vi "Test Message in Ressult without Description.vi"(8 "error in (no error)":errorcluster, 11 "Compare Assertion Test In":refnum<class "Compare Assertion Test.lvclass">) -> (0 "error out":errorcluster, 3 "Compare Assertion Test Out":refnum<class "Compare Assertion Test.lvclass">)   [LabVIEW 2020, in "LUnit Tests.lvlib" / "Compare Assertion Test.lvclass"]
uses:
  Compare Assertion Test.lvclass
  Compare Assertion Test.lvclass/Compare Assertion Test.ctl
  Test Dummys/Test Case Test Double/Test Case Test Double.lvclass
  <vilib>/Astemes/LUnit/Test Case.lvclass
  C:/Program Files (x86)/National Instruments/LabVIEW 2020/vi.lib/Astemes/LUnit/Test Case.lvclass
  C:/Git/astemes-lunit/tests/Compare Assertion Test/Compare Assertion Test.lvclass
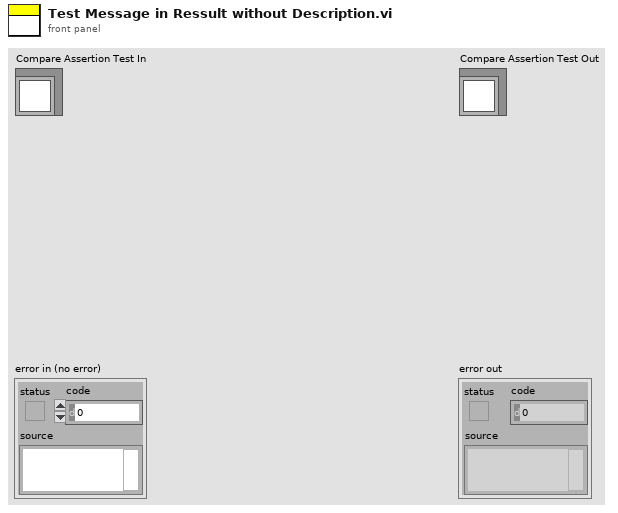
[diagram p1: front panel]
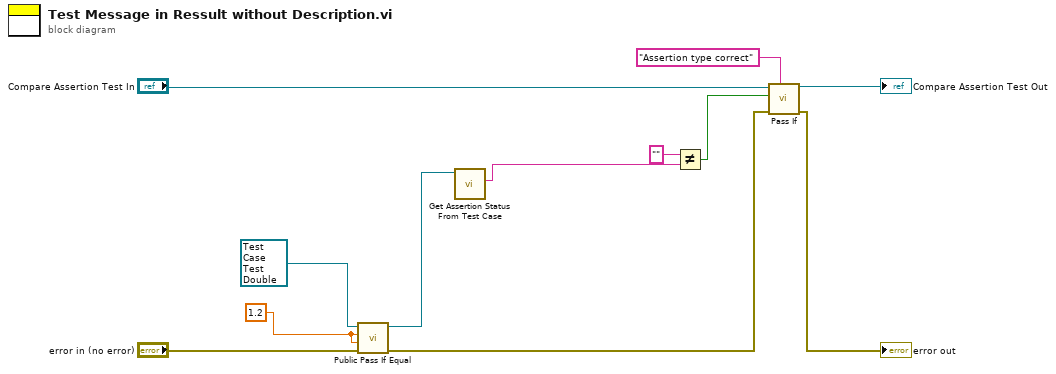
[diagram p0: block diagram]
diagram:
  w3 = 1.2
  n1 = call "Public Pass If Equal.vi"("error in (no error)"="error in (no error)", "Actual"=w3, "Expected"=w3, "Test Case Test Double in"=refnum<class "Test Case Test Double.lvclass"> refnum ("Test Case Test Double.lvclass")) -> ("error out"=w9:errorcluster, "Test Case Test Double out"=w8:refnum<class "Test Case Test Double.lvclass">)  [unwired: 6 in]
  n2 = call "Get Assertion Status From Test Case.vi"("Test Case Test Double in"=w8) -> ("Message"=w2:string)  [unwired: 9 in, 1 out]
  n3 = Not Equal?(x="", y=w2) -> (x != y?=w11:bool)
  n4 = call <vilib>:"Pass If.vi"("Description"="Assertion type correct", "error in (no error)"=w9, "Pass?"=w11, "LUnit Test Case In"="Compare Assertion Test In") -> ("error out"=→"error out":errorcluster, "LUnit Test Case Out"=→"Compare Assertion Test Out":refnum<class "Compare Assertion Test.lvclass">)  [unwired: 6 in]
